vi "who is clever(visible and invisible.vi"() -> ()   [LabVIEW 2018]
panel:
  in  "stop":bool
  in  "yes":bool
  in  "no":bool
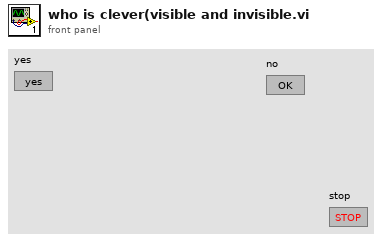
[diagram p1: front panel]
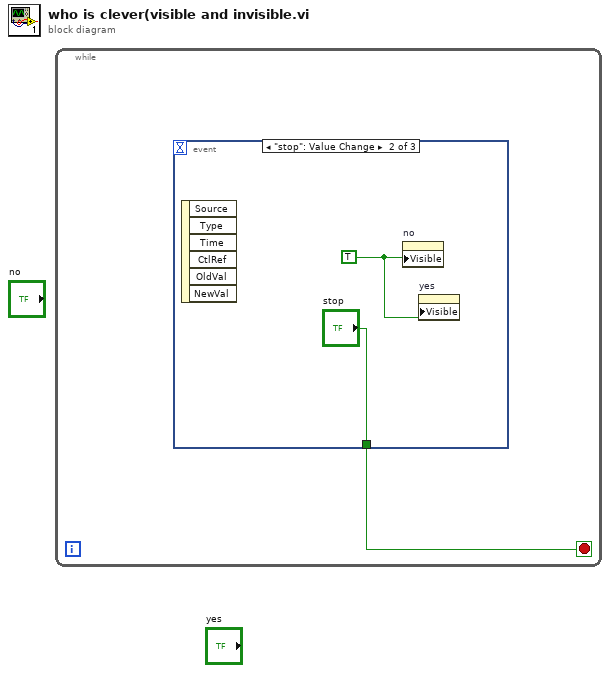
[diagram p0: block diagram]
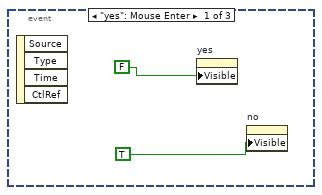
[diagram p2: hidden frame]
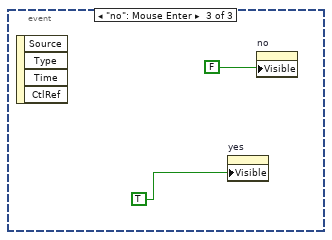
[diagram p3: hidden frame]
diagram:
  n1 = while {
    stop <- w1 stop-if-true
    n2 = event shown="[1] \"stop\": Value Change" {
      selector: _ -> [_ _ _]
      dyn-events: _ -> [_ _ _]
      timeout: _ -> [_ _ _]
      tunnel: [_ "stop" _] -> w1
      event "yes": Mouse Enter {
        n3 = event-data() -> ()  [unwired: 1 in, 4 out]
        n4 = property on="yes" class="Bool"("Visible"=FALSE) -> ()  [unwired: 2 in, 2 out]
        n5 = property on="no" class="Bool"("Visible"=TRUE) -> ()  [unwired: 2 in, 2 out]
      }
      event "stop": Value Change {
        w4 = TRUE
        n6 = event-data() -> ()  [unwired: 1 in, 6 out]
        n7 = property on="no" class="Bool"("Visible"=w4) -> ()  [unwired: 2 in, 2 out]
        n8 = property on="yes" class="Bool"("Visible"=w4) -> ()  [unwired: 2 in, 2 out]
      }
      event "no": Mouse Enter {
        n9 = event-data() -> ()  [unwired: 1 in, 4 out]
        n10 = property on="yes" class="Bool"("Visible"=TRUE) -> ()  [unwired: 2 in, 2 out]
        n11 = property on="no" class="Bool"("Visible"=FALSE) -> ()  [unwired: 2 in, 2 out]
      }
    }
  }
